vi "Second step for time diagram.vi"(7 "Массив со значениями задержек":i32[](array[numeric]), 8 "left 1 vertical (1 или 0)":i32[](array[numeric]), 9 "left 1 vertical (время)":i32[](array[numeric]), 10 "left 1 gorizontal(1 или 0)":i32[](array[numeric]), 11 "left 1 gorizontal(время)":i32[](array[numeric])) -> (0 "right vertical(0 или 1)":i32[](array[numeric]), 1 "right vertical (время)":i32[](array[numeric]), 2 "right gorizontal(0 или 1)":i32[](array[numeric]), 3 "right gorizontal(время)":i32[](array[numeric]), 5 "Тактовая диаграмма":cluster{i32[], i32[]}[](graph))   [LabVIEW 2012]
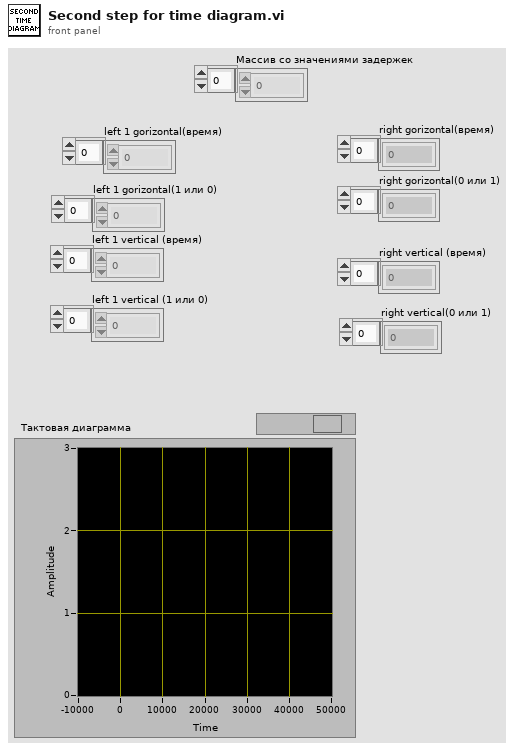
[diagram p1: front panel]
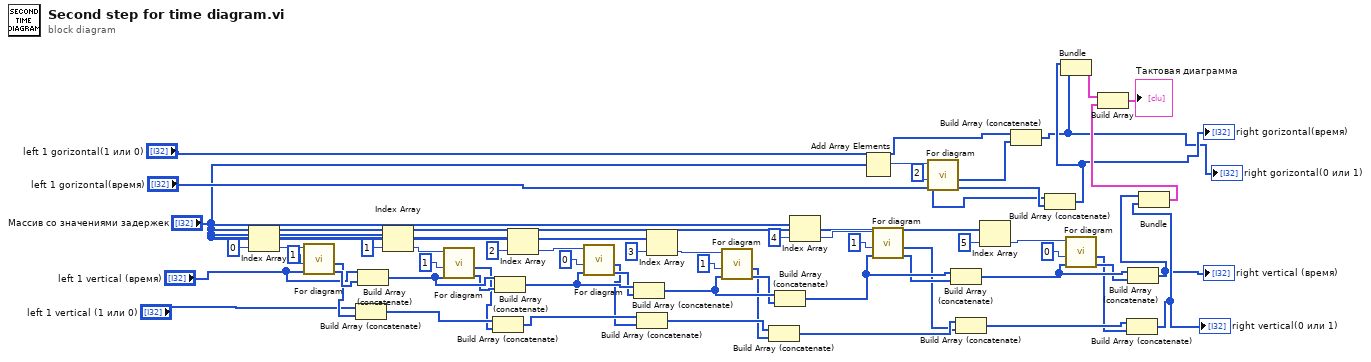
[diagram p0: block diagram]
diagram:
  n1 = Index Array(array="Массив со значениями задержек", index=0) -> (element=w14:i32)
  n2 = call "For diagram.vi"("Предыдущий массив"="left 1 vertical (время)", "Номер импульса"=1, "Время в милисикундах"=w14) -> ("Кол-во точек (время в милисек)"=w46:i32[], "Номер импульса (0 или 1)"=w45:i32[])  [unwired: 7 in]
  n3 = Build Array (concatenate)("left 1 vertical (1 или 0)", w45) -> (w43:i32[])
  n4 = Build Array (concatenate)("left 1 vertical (время)", w46) -> (w44:i32[])
  n5 = Index Array(array="Массив со значениями задержек", index=1) -> (element=w4:i32)
  n6 = call "For diagram.vi"("Предыдущий массив"=w44, "Номер импульса"=1, "Время в милисикундах"=w4) -> ("Кол-во точек (время в милисек)"=w26:i32[], "Номер импульса (0 или 1)"=w25:i32[])  [unwired: 7 in]
  n7 = Build Array (concatenate)(w43, w25) -> (w42:i32[])
  n8 = Build Array (concatenate)(w44, w26) -> (w38:i32[])
  n9 = Index Array(array="Массив со значениями задержек", index=2) -> (element=w5:i32)
  n10 = call "For diagram.vi"("Предыдущий массив"=w38, "Номер импульса"=0, "Время в милисикундах"=w5) -> ("Кол-во точек (время в милисек)"=w28:i32[], "Номер импульса (0 или 1)"=w27:i32[])  [unwired: 7 in]
  n11 = Build Array (concatenate)(w38, w28) -> (w37:i32[])
  n12 = Build Array (concatenate)(w42, w27) -> (w41:i32[])
  n13 = Index Array(array="Массив со значениями задержек", index=3) -> (element=w6:i32)
  n14 = call "For diagram.vi"("Предыдущий массив"=w37, "Номер импульса"=1, "Время в милисикундах"=w6) -> ("Кол-во точек (время в милисек)"=w30:i32[], "Номер импульса (0 или 1)"=w29:i32[])  [unwired: 7 in]
  n15 = Build Array (concatenate)(w41, w29) -> (w40:i32[])
  n16 = Build Array (concatenate)(w37, w30) -> (w36:i32[])
  n17 = Index Array(array="Массив со значениями задержек", index=4) -> (element=w7:i32)
  n18 = Add Array Elements(numeric array="Массив со значениями задержек") -> (sum=w55:i32)
  n19 = call "For diagram.vi"("Предыдущий массив"=w36, "Номер импульса"=1, "Время в милисикундах"=w7) -> ("Кол-во точек (время в милисек)"=w32:i32[], "Номер импульса (0 или 1)"=w31:i32[])  [unwired: 7 in]
  n20 = call "For diagram.vi"("Предыдущий массив"="left 1 gorizontal(время)", "Номер импульса"=2, "Время в милисикундах"=w55) -> ("Кол-во точек (время в милисек)"=w54:i32[], "Номер импульса (0 или 1)"=w53:i32[])  [unwired: 7 in]
  n21 = Build Array (concatenate)(w36, w32) -> (w35:i32[])
  n22 = Build Array (concatenate)(w40, w31) -> (w39:i32[])
  n23 = Index Array(array="Массив со значениями задержек", index=5) -> (element=w8:i32)
  n24 = Build Array (concatenate)("left 1 gorizontal(1 или 0)", w53) -> (w1:i32[])
  "right gorizontal(0 или 1)" <- w1
  n25 = Build Array (concatenate)("left 1 gorizontal(время)", w54) -> (w2:i32[])
  "right gorizontal(время)" <- w2
  n26 = Bundle(w2, w1) -> (w24:cluster{i32[], i32[]})  [unwired: 1 in]
  n27 = call "For diagram.vi"("Предыдущий массив"=w35, "Номер импульса"=0, "Время в милисикундах"=w8) -> ("Кол-во точек (время в милисек)"=w34:i32[], "Номер импульса (0 или 1)"=w33:i32[])  [unwired: 7 in]
  n28 = Build Array (concatenate)(w39, w33) -> (w23:i32[])
  "right vertical(0 или 1)" <- w23
  n29 = Build Array (concatenate)(w35, w34) -> (w20:i32[])
  "right vertical (время)" <- w20
  n30 = Bundle(w20, w23) -> (w22:cluster{i32[], i32[]})  [unwired: 1 in]
  n31 = Build Array(w24, w22) -> (→"Тактовая диаграмма":cluster{i32[], i32[]}[])
